vi "test rotate Array.vi"() -> ()   [LabVIEW 2019]
panel:
  out "sum":dbl
  in  "Array size":i32=3600
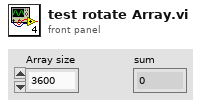
[diagram p1: front panel]
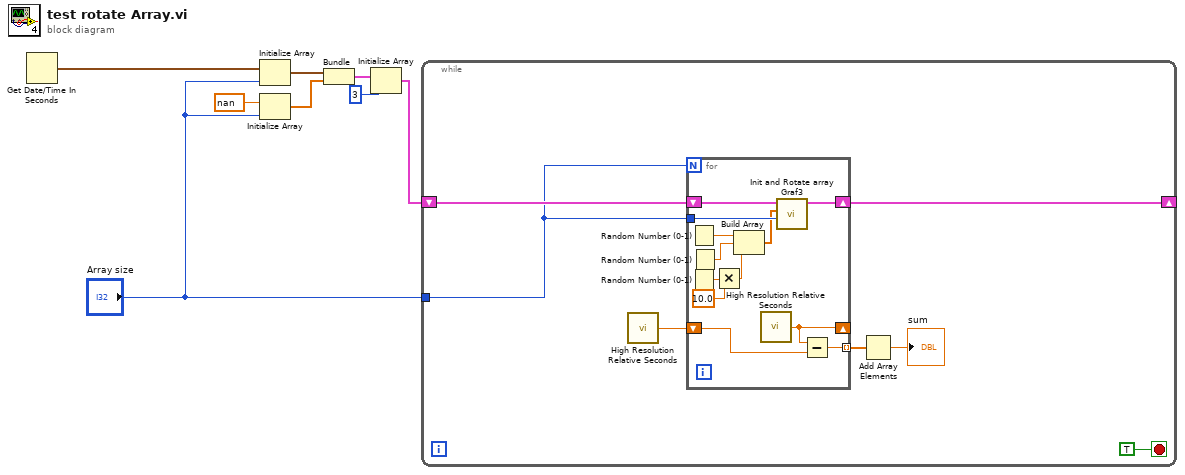
[diagram p0: block diagram]
diagram:
  n1 = Get Date/Time In Seconds() -> (seconds since 1Jan1904=w6:timestamp)
  n2 = Initialize Array(w6, "Array size") -> (w5:timestamp[])
  n3 = Initialize Array(nan ("PV"), "Array size") -> (w4:dbl[])
  n4 = Bundle(w5, w4) -> (w3:cluster{timestamp[], dbl[]})  [unwired: 1 in]
  n5 = Initialize Array(w3, 3 ("dimension size")) -> (w1:cluster{timestamp[], dbl[]}[])
  n6 = while {
    shift-right: [w14] -> _
    shift-left: w1 -> [w13]
    tunnel: "Array size" -> [w11]
    stop <- TRUE stop-if-true
    n7 = call <vilib>:"High Resolution Relative Seconds.vi"() -> ("relative seconds"=w12:dbl)
    n8 = for {
      N: w11 -> [_]
      tunnel: w11 -> [w25]
      shift-right: [w27] -> w14
      shift-left: w13 -> [w26]
      shift-right: [w17] -> _
      shift-left: w12 -> [w18]
      tunnel: [w16] -> w10 mode=indexing
      n9 = Random Number (0-1)() -> (number: 0 to 1=w23:dbl)
      n10 = Random Number (0-1)() -> (number: 0 to 1=w20:dbl)
      n11 = Random Number (0-1)() -> (number: 0 to 1=w22:dbl)
      n12 = Multiply(x=w20, y=10.0) -> (x*y=w21:dbl)
      n13 = Build Array(w23, w22, w21) -> (w24:dbl[])
      n14 = call <vilib>:"High Resolution Relative Seconds.vi"() -> ("relative seconds"=w17:dbl)
      n15 = call "Init and Rotate array Graf3.vi"("Array size"=w25, "PV"=w24, "XY Graf in"=w26) -> ("XY Graf out"=w27:cluster{"time stamp":timestamp[], "PV":dbl[]}[])  [unwired: 8 in]
      n16 = Subtract(x=w17, y=w18) -> (x-y=w16:dbl)
    }
    n17 = Add Array Elements(numeric array=w10) -> (sum=→"sum":dbl)
  }
